vi "BGA244_meas.vi"(8 "error in":errorcluster, 11 "VISA in":refnum<visa-resource-name>) -> (0 "error out":errorcluster, 1 "ratio2":dbl, 2 "ratio1":dbl, 3 "VISA out":refnum<visa-resource-name>, 4 "status":bool)   [LabVIEW 2019]
panel:
  out "string 2":string
  out "string 1":string
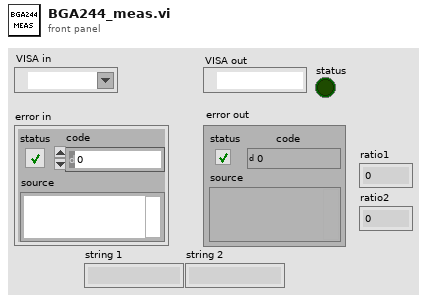
[diagram p1: front panel]
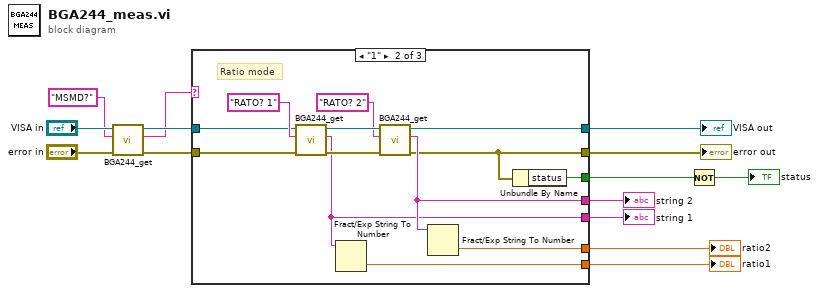
[diagram p0: block diagram]
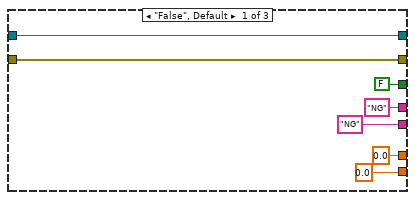
[diagram p2: hidden frame]
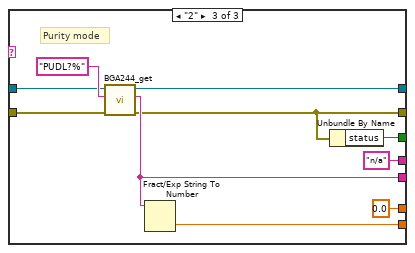
[diagram p3: hidden frame]
diagram:
  n1 = call "BGA244_get.vi"("error in"="error in", "string in"="MSMD?", "VISA in"="VISA in") -> ("error out"=w11:errorcluster, "string out"=w6:string, "VISA out"=w10:refnum<visa-resource-name>)  [unwired: 6 in]
  n2 = case shown="\"1\"" w6 {
    tunnel: [w21 w32 w41] -> w14
    tunnel: [w20 w22 w35] -> w13
    tunnel: w11 -> [w20 w29 w42]
    tunnel: w10 -> [w21 w28 w43]
    tunnel: [0.0 w27 0.0] -> w5
    tunnel: [0.0 w26 w38] -> w4
    tunnel: ["NG" ("string out") w25 "n/a" ("string out")] -> w3
    tunnel: ["NG" ("string out") w24 w40] -> w2
    tunnel: [FALSE ("status") w23 w36] -> w1
    frame "False", Default {
    }
    frame "1" {
      # "Ratio mode"
      n3 = call "BGA244_get.vi"("error in"=w29, "string in"="RATO? 1" ("string"), "VISA in"=w28) -> ("error out"=w31:errorcluster, "string out"=w24:string, "VISA out"=w33:refnum<visa-resource-name>)  [unwired: 6 in]
      n4 = Fract/Exp String To Number(string=w24) -> (number=w26:dbl)  [unwired: 3 in, 1 out]
      n5 = call "BGA244_get.vi"("error in"=w31, "string in"="RATO? 2" ("string"), "VISA in"=w33) -> ("error out"=w22:errorcluster, "string out"=w25:string, "VISA out"=w32:refnum<visa-resource-name>)  [unwired: 6 in]
      n6 = Fract/Exp String To Number(string=w25) -> (number=w27:dbl)  [unwired: 3 in, 1 out]
      n7 = Unbundle By Name(w22) -> ("status"=w23:bool)
    }
    frame "2" {
      # "Purity mode"
      n8 = call "BGA244_get.vi"("error in"=w42, "string in"="PUDL?%" ("string"), "VISA in"=w43) -> ("error out"=w35:errorcluster, "string out"=w40:string, "VISA out"=w41:refnum<visa-resource-name>)  [unwired: 6 in]
      n9 = Fract/Exp String To Number(string=w40) -> (number=w38:dbl)  [unwired: 3 in, 1 out]
      n10 = Unbundle By Name(w35) -> ("status"=w36:bool)
    }
  }
  "VISA out" <- w14
  "error out" <- w13
  "ratio1" <- w4
  "ratio2" <- w5
  "string 2" <- w3
  "string 1" <- w2
  n11 = Not(x=w1) -> (.not. x?=→"status":bool)
